vi "setHorizontalSettingsToHW.vi"(8 "error in (no error)":errorcluster, 10 "Horizontal":T1 {"time_window" step=1000000.0 format="%.2p"}, 11 "TektronixDPO in":refnum<class "TektronixDPO.lvclass">) -> (0 "error out":errorcluster, 3 "TektronixDPO out":refnum<class "TektronixDPO.lvclass">)   [LabVIEW 2013, in "TektronixDPO.lvclass"]
doc: "Send the horizontal configuration to the physical device"
uses:
  TektronixDPO.lvclass
  TypeDefs/Horizontal.ctl
  shared/Typdefs/Choice77.ctl
  TektronixDPO.lvclass/TektronixDPO.ctl
  Tektronix DPO MSO 2000 4000 Series/Tektronix DPO MSO 2000 4000 Series.lvlib
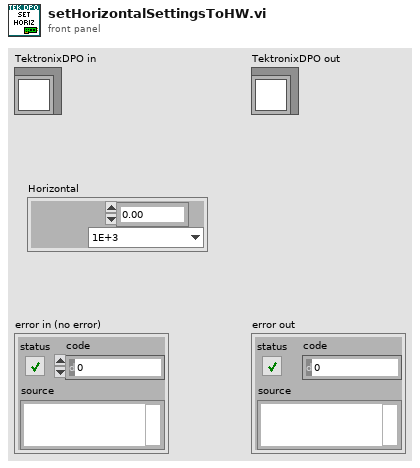
[diagram p1: front panel]
types:
  T1 = typedef "Horizontal.ctl" = cluster{"time_window":dbl, "resolution":T2}
  T2 = typedef "Choice77.ctl" = enum16{"1E+3", "10E+3", "100E+3", "1E+6", "5E+6", "10E+6"}
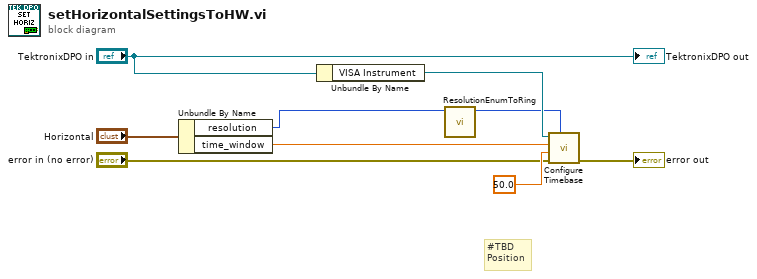
[diagram p0: block diagram]
diagram:
  # "#TBD\nPosition"
  n1 = Unbundle By Name("Horizontal") -> ("resolution"=w3:T2, "time_window"=w7:dbl)
  n2 = Unbundle By Name("TektronixDPO in") -> ("VISA Instrument"=w8:refnum<visa-resource-name>)
  n3 = call "ResolutionEnumToRing.vi"("resolution"=w3) -> ("Resolutinon"=w4:u32)  [unwired: 10 in]
  n4 = call "Configure Timebase.vi"("Record Length (10: 10k points)"=w4, "error in (no error)"="error in (no error)", "Position (10 %)"=50.0, "Timebase (0.0005 s)"=w7, "VISA resource name"=w8) -> ("error out"=→"error out":errorcluster)  [unwired: 5 in, 1 out]
  "TektronixDPO out" <- "TektronixDPO in"
